vi "Data_Queue_Open.vi"(8 "error in (no error)":errorcluster, 11 "Ref in":T1 {"TS Parameter"."FCA" format="%01d"; "TS Parameter"."Target" min=1 max=100000; "TS Parameter"."PokaYoke" min=0 max=1}) -> (0 "error out":errorcluster, 3 "Ref out":T1 {"TS Parameter"."FCA" format="%01d"; "TS Parameter"."Target" min=1 max=100000; "TS Parameter"."PokaYoke" min=0 max=1})   [LabVIEW 2020]
uses:
  Controls/TD SQL.ctl
  <vilib>/addons/database/Connection.llb/Conn ObjectReference.ctl
  Controls/WIP_State.ctl
  Controls/TS_Parameter.ctl
  <vilib>/addons/database/NI_Database_API.lvlib
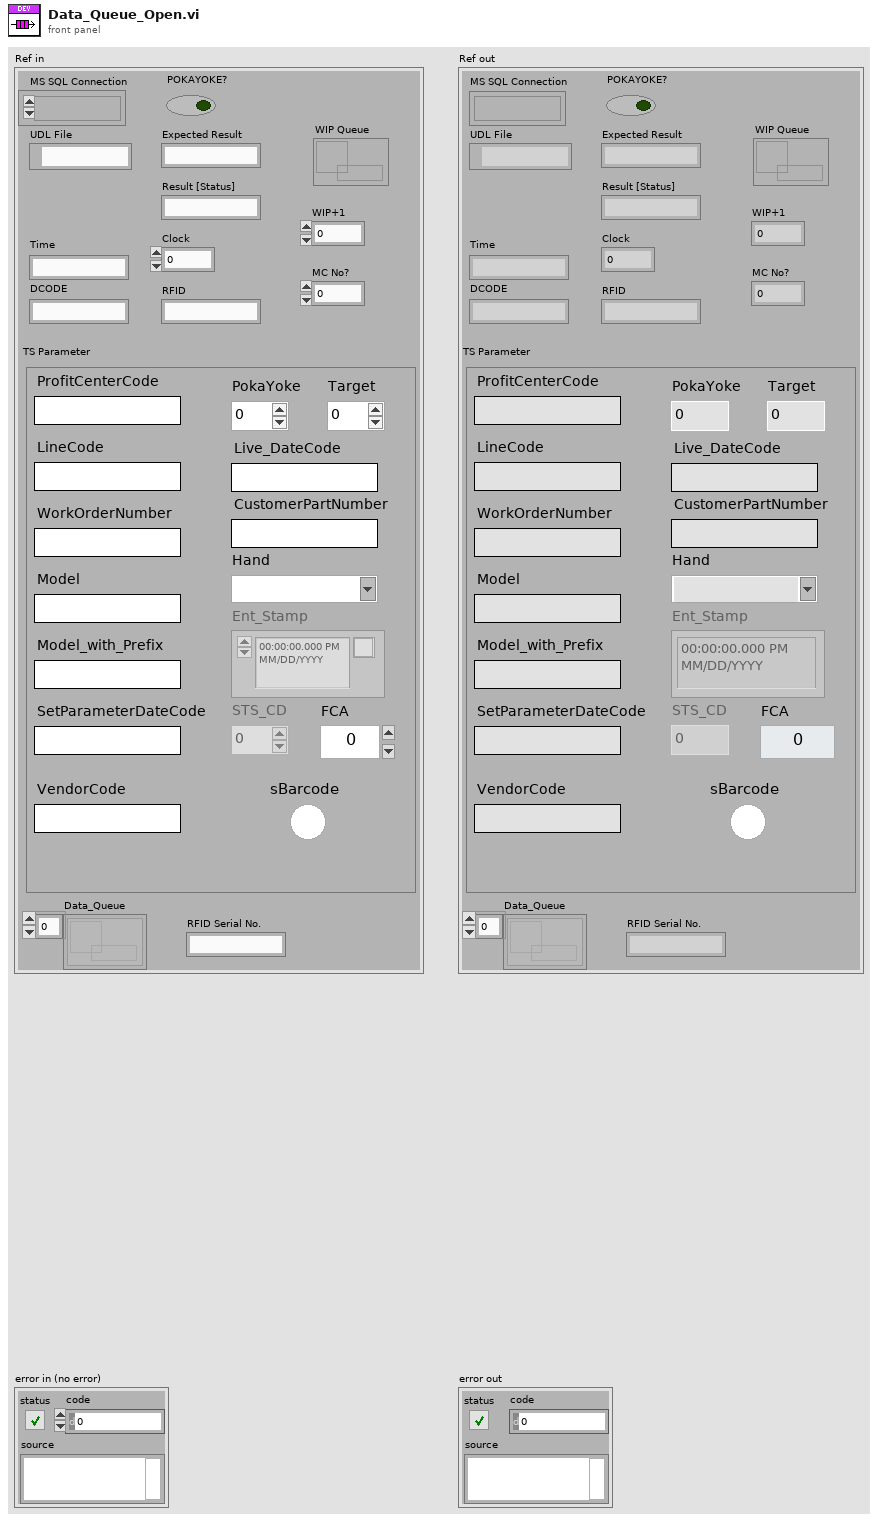
[diagram p1: front panel]
types:
  T1 = typedef "TD SQL.ctl" = cluster{"MS SQL Connection":T2, "UDL File":path, "Time":string, "DCODE":string, "WIP+1":i64, "MC No?":i32, "POKAYOKE?":bool, "Expected Result":string, "Result [Status]":string, "Clock":dbl, "RFID":string, "WIP Queue":refnum<queue>, "TS Parameter":T3, "Data_Queue":refnum<queue>[], "RFID Serial No.":string}
  T2 = typedef "NI_Database_API.lvlib/Conn ObjectReference.ctl" = refnum<k1>
  T3 = typedef "TS_Parameter.ctl" = cluster{"ProfitCenterCode":string, "LineCode":string, "WorkOrderNumber":string, "Model":string, "Model_with_Prefix":string, "VendorCode":string, "SetParameterDateCode":string, "PokaYoke":i32, "Target":i32, "Live_DateCode":string, "CustomerPartNumber":string, "Hand":string, "sBarcode":bool, "FCA":i32, "Ent_Stamp":timestamp, "STS_CD":dbl}
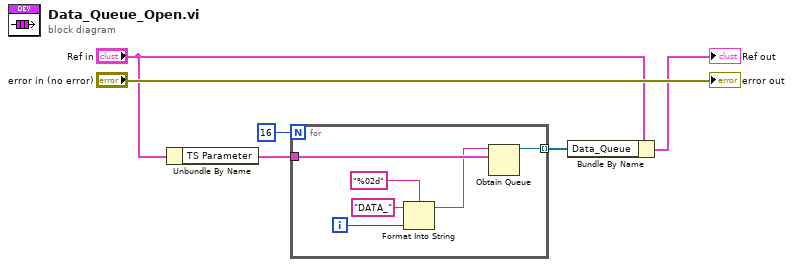
[diagram p0: block diagram]
diagram:
  n1 = Unbundle By Name("Ref in") -> ("TS Parameter"=w3:T3)
  n2 = for {
    N: 16 -> [_]
    tunnel: w3 -> [w9]
    tunnel: [w7] -> w1 mode=indexing
    i -> [w12]
    n3 = Format Into String(format string="%02d", initial string="DATA_", w12) -> (resulting string=w8:string)  [unwired: 1 in, 1 out]
    n4 = Obtain Queue(name (unnamed)=w8, element data type=w9) -> (queue out=w7:refnum<queue>)  [unwired: 3 in, 2 out]
  }
  n5 = Bundle By Name(cluster="Ref in", "Data_Queue"=w1) -> (→"Ref out":T1)
  "error out" <- "error in (no error)"
